vi "Acquire Data.vi"(8 "error in (no error)":errorcluster, 11 "Configuration Settings":T1={"Signal type"=enum."Sine Wave", "Amplitude"=1.0, "Offset"=0.0, "Amplitude 2"=1.0, "Frequency"=10.0} {"Frequency" format="%0.2p"; "Amplitude 2" format="%.2p"; "Offset" format="%0.2p"; "Amplitude" format="%0.2p"}) -> (0 "error out":errorcluster, 3 "Data Out":dbl[](array[numeric]))   [LabVIEW 2022 SP3]
uses:
  controls/Configuration Settings.ctl
  <vilib>/measure/NI_MABase.lvlib
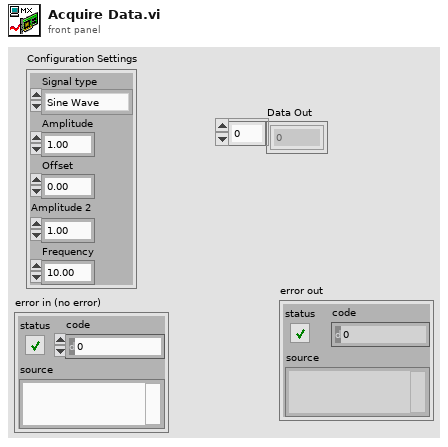
[diagram p1: front panel]
types:
  T1 = typedef "Configuration Settings.ctl" = cluster{"Signal type":enum16{"Sine Wave", "Triangle Wave", "Square Wave", "Sawtooth Wave"}, "Amplitude":dbl, "Offset":dbl, "Amplitude 2":dbl, "Frequency":dbl}
  T2 = enum16{"Sine Wave", "Triangle Wave", "Square Wave", "Sawtooth Wave"}
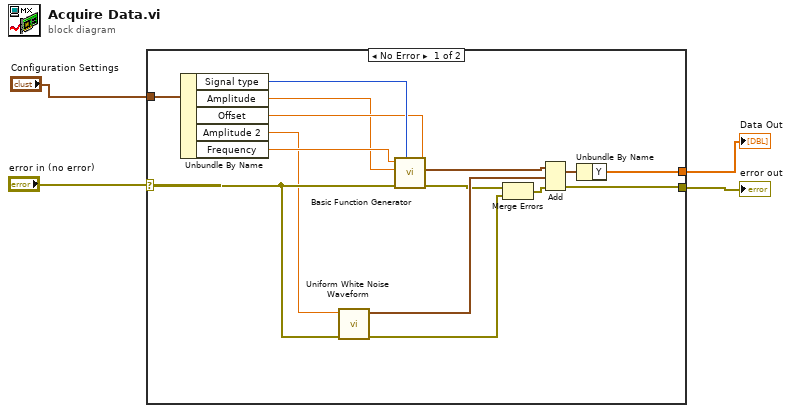
[diagram p0: block diagram]
diagram:
  n1 = case shown="No Error" "error in (no error)" {
    selector: "error in (no error)" -> [w14 w20]
    tunnel: [w17 w20] -> w3
    tunnel: [w15 _] -> w2
    tunnel: "Configuration Settings" -> [w10 _]
    frame No Error {
      n2 = Unbundle By Name(w10) -> ("Signal type"=w9:T2, "Amplitude"=w5:dbl, "Offset"=w8:dbl, "Amplitude 2"=w6:dbl, "Frequency"=w7:dbl)
      n3 = call <vilib>:"Uniform White Noise Waveform.vi"("error in (no error)"=w14, "amplitude"=w6) -> ("error out"=w12:errorcluster, "signal out"=w18:waveform(dbl))  [unwired: 8 in]
      n4 = call <vilib>:"Basic Function Generator.vi"("offset"=w8, "signal type"=w9, "error in (no error)"=w14, "amplitude"=w5, "frequency"=w7) -> ("error out"=w13:errorcluster, "signal out"=w19:waveform(dbl))  [unwired: 4 in, 1 out]
      n5 = Merge Errors(w13, w12) -> (w11:errorcluster)
      n6 = Add(1:w18, 2:w19, 4:w11) -> (0:w16:waveform(dbl), 3:w17:errorcluster)
      n7 = Unbundle By Name(w16) -> ("Y"=w15:dbl[])
    }
    frame Error {
    }
  }
  "error out" <- w3
  "Data Out" <- w2
